vi "Speed of sound VI.vi"() -> ()   [LabVIEW 2021]
uses:
  <vilib>/express/express arith-compare/Formula/XNode/ExpressFormulaBlockNode.xnode
panel:
  out "Result":dbl
  in  "T temp in F":dbl
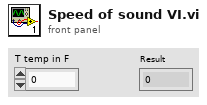
[diagram p1: front panel]
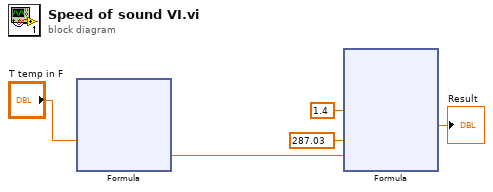
[diagram p0: block diagram]
diagram:
  n1 = xnode "Formula"("temp"="T temp in F") -> ("Result"=w1:dbl)  [unwired: 1 in, 1 out]
  n2 = xnode "Formula"("v"=1.4, "R"=287.03, "T"=w1) -> ("Result"=→"Result":dbl)  [unwired: 1 in, 1 out]
